vi "Obtain I2C.vi"(4 "SDA GPIO":T2=-1, 5 "Purpose (\"I2C\")":string="I2C", 6 "SCL GPIO":T2=-1, 7 "I2C #":T1=-1, 8 "error in (no error)":errorcluster, 10 "Baud":u32=400000 format="%.0p", 11 "Session in":refnum<class "Session.lvclass">) -> (0 "error out":errorcluster, 2 "I2C":refnum<class "I2C.lvclass">, 3 "Session out":refnum<class "Session.lvclass">)   [LabVIEW 2020, in "CTI.lvlib" / "Session.lvclass"]
uses:
  Session.lvclass
  GPIO Number.ctl
  I2C Number.ctl
  I2C/I2C.lvclass
  I2C Pins.ctl
  Session.lvclass/Session.ctl
  a62e29e6-9d1f-431a-a6fd-f8ae5f19d440.vi
  a62e29e6-9d1f-431a-a6fd-f8ae5f19d440.vi/1ebac61a-bcc0-4be5-9ea8-8faf7576f3c5.vi
  Is Full Errors.vi
  Check Errors.vi
  CTI.lvlib
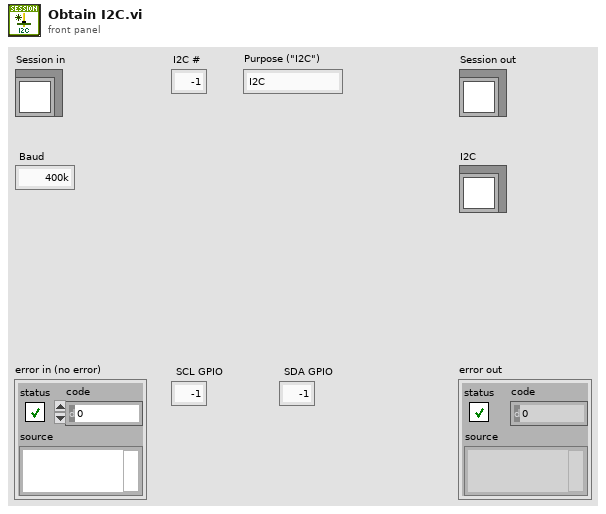
[diagram p1: front panel]
types:
  T1 = typedef "CTI.lvlib/I2C Number.ctl" = i8
  T2 = typedef "CTI.lvlib/GPIO Number.ctl" = i8
  T3 = typedef "CTI.lvlib/I2C Pins.ctl" = cluster{"SDA GPIO":T2, "SCL GPIO":T2}
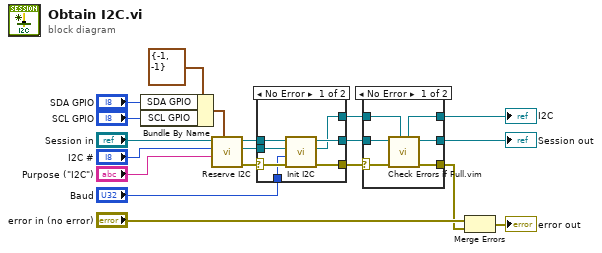
[diagram p0: block diagram]
diagram:
  n1 = Bundle By Name(cluster=T3 {"SDA GPIO"=-1, "SCL GPIO"=-1} ("I2C Pins"), "SDA GPIO"="SDA GPIO", "SCL GPIO"="SCL GPIO") -> (w15:T3)
  n2 = call "Reserve I2C.vi"("I2C Pins"=w15, "Purpose"="Purpose (\"I2C\")", "I2C #"="I2C #", "Session in"="Session in") -> ("error out"=w12:errorcluster, "I2C"=w10:refnum<class "I2C.lvclass">, "Session out"=w11:refnum<class "Session.lvclass">)  [unwired: 5 in]
  n3 = case shown="No Error" w12 {
    selector: w12 -> [w24 w28]
    tunnel: w11 -> [w26 w27]
    tunnel: w10 -> [w25 _]
    tunnel: "Baud" -> [w23 _]
    tunnel: [w22 w27] -> w7
    tunnel: [w21 w28] -> w8
    tunnel: [w20 _] -> w6
    frame No Error {
      n4 = call-dynamic "Init I2C.vi"("error in (no error)"=w24, "Baud"=w23, "I2C In"=w25, "Session in"=w26) -> ("error out"=w21:errorcluster, "I2C"=w20:refnum<class "I2C.lvclass">, "Session out"=w22:refnum<class "Session.lvclass">)  [unwired: 5 in]
    }
    frame Error {
    }
  }
  n5 = case shown="No Error" w8 {
    selector: w8 -> [w33 w35]
    tunnel: w7 -> [w34 w36]
    tunnel: w6 -> [w32 _]
    tunnel: [w31 _] -> w5
    tunnel: [w30 w36] -> w4
    tunnel: [w29 w35] -> w2
    frame No Error {
      n6 = call "Check Errors if Full.vim"("Resource In"=w32, "error in (no error)"=w33, "Session in"=w34) -> ("error out"=w29:errorcluster, "Session out"=w30:refnum<class "Session.lvclass">, "Resource"=w31:refnum<class "I2C.lvclass">)  [unwired: 6 in]
    }
    frame Error {
    }
  }
  "Session out" <- w4
  "I2C" <- w5
  n7 = Merge Errors("error in (no error)", w2) -> (→"error out":errorcluster)
